vi "SafeSendCommand.vi"(6 "error in":errorcluster, 8 "Parameter":sgl, 9 "Command #":u8=8, 10 "Address #":u8, 11 "VISA resource name":refnum<visa-resource-name>) -> (0 "error out":errorcluster, 1 "Raw Response":string, 2 "Value":dbl, 3 "VISA resource name out":refnum<visa-resource-name>)   [LabVIEW 2020, in "driver_flodx_rtd.lvlib"]
doc: "Sends a 'Safe' command, \nFirst a message is sent given the address, command #, and parameter. The FloDx then responds and that \nresponse is validated. If the message is valid, the value returned is outputted. If not multiple errors are thrown."
uses:
  <instrlib>/RxnRover/FloDx RTD Driver/driver_flodx_rtd.lvlib
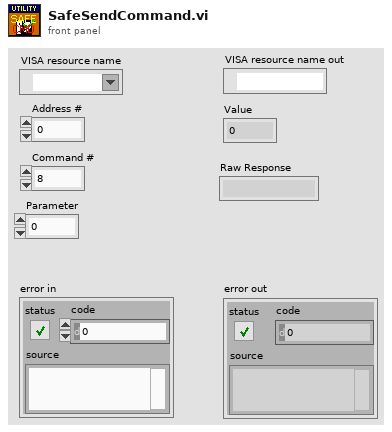
[diagram p1: front panel]
types:
  T1 = cluster{"Address":u32, "Command":u32, "Value":dbl, "Error Code":u32}
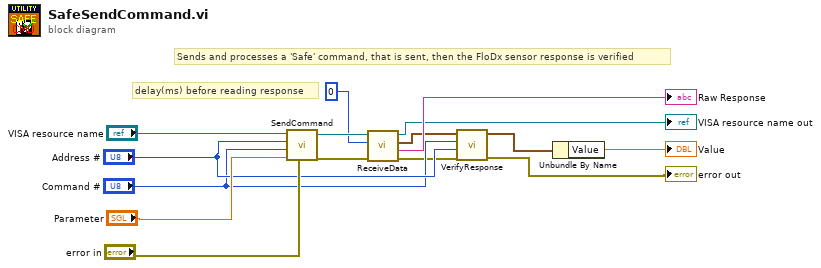
[diagram p0: block diagram]
diagram:
  # "delay(ms) before reading response"
  # "Sends and processes a 'Safe' command, that is sent, then the FloDx sensor response is verified"
  n1 = call <instrlib>:"SendCommand.vi"("error in"="error in", "Parameter"="Parameter", "Command"="Command #", "Address"="Address #", "VISA resource name"="VISA resource name") -> ("error out"=w13:errorcluster, "VISA resource name out"=w15:refnum<visa-resource-name>)  [unwired: 4 in, 1 out]
  n2 = call <instrlib>:"ReceiveData.vi"("error in (no error)"=w13, "Delay before read (ms)"=u32 0, "VISA resource name"=w15) -> ("error out"=w3:errorcluster, "Raw Response"=→"Raw Response":string, "Recieved Data"=w4:T1, "VISA resource name out"=→"VISA resource name out":refnum<visa-resource-name>)  [unwired: 4 in, 1 out]
  n3 = call <instrlib>:"VerifyResponse.vi"("error in"=w3, "Address #"="Address #", "Command #"="Command #", "Data In"=w4) -> ("error out"=→"error out":errorcluster, "Data out"=w2:T1)  [unwired: 6 in]
  n4 = Unbundle By Name(w2) -> ("Value"=→"Value":dbl)
